vi "String - XML 2-Byte Decoding.vi"(0 "Number In (3-Bytes -24bits)":i32 format="%x", 3 "Error In":errorcluster) -> (7 "Output (\\ Format)":string, 8 "Output 16bits":i16=-30048 format="%04x", 10 "Error Out":errorcluster)   [LabVIEW 2013]
panel:
  out "YYYYYY  (6bits) 3":i32=2560 format="%024b"
  in  "Use Number In":bool=TRUE
  out "16bits":u32 format="%x"
  in  "String In (3-Byte Width)":string
  out "Swapped Bytes":i16=21152 format="%x"
  out "ZZZZZZ  (6bits) 3":i32=32 format="%024b"
  out "YYYYYY  (6bits) 2":i32=2560 format="%024b"
  out "XXXX  (4bits) 1":i32=327680 format="%024b"
  out "Output  (24bits)":i32=15043232 format="%024b"
  out "Input (21bits)":u32=21152 format="%021b"
  # "Otherwise, if the code point is less than 10000 (16) output the bitwise inclusive OR of bits 13 through 16 with EO16"
  # "E696 B0"
  # "B065"
  # "E58A A0"
  # "A052"
  # "E59DA1"
  # "6157"
  # "°e RaW"
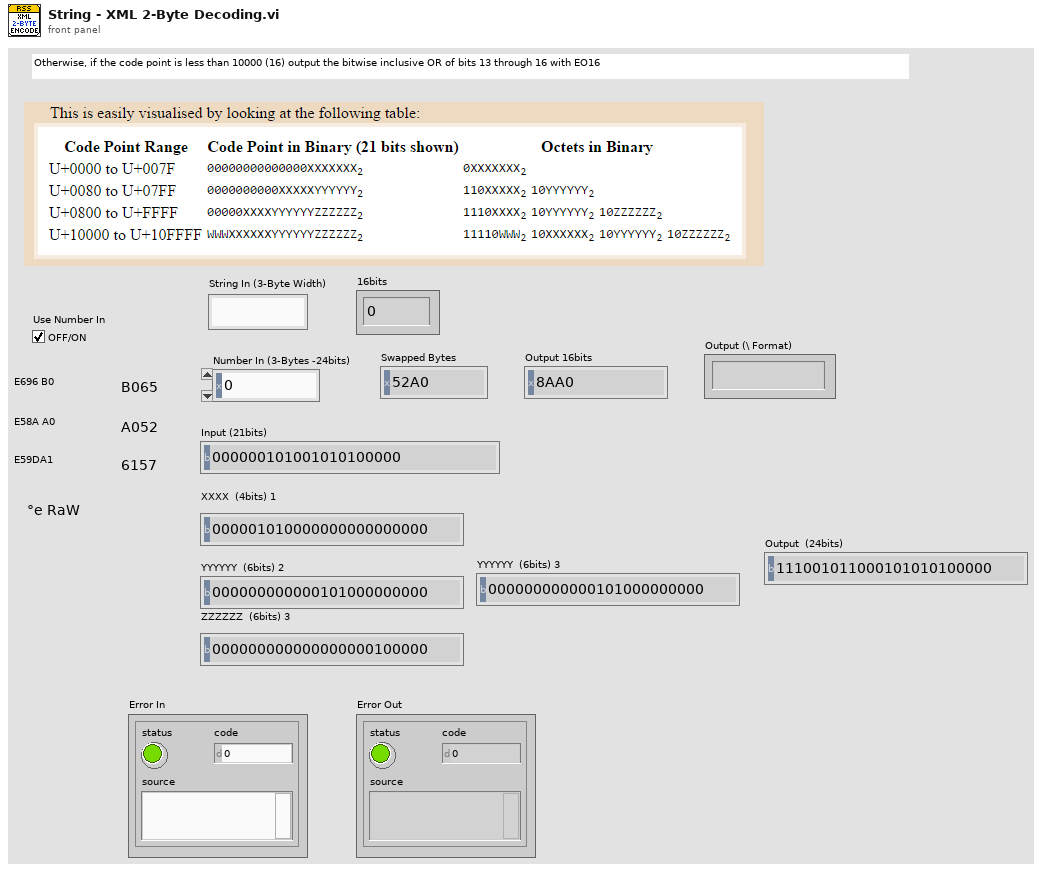
[diagram p1: front panel]
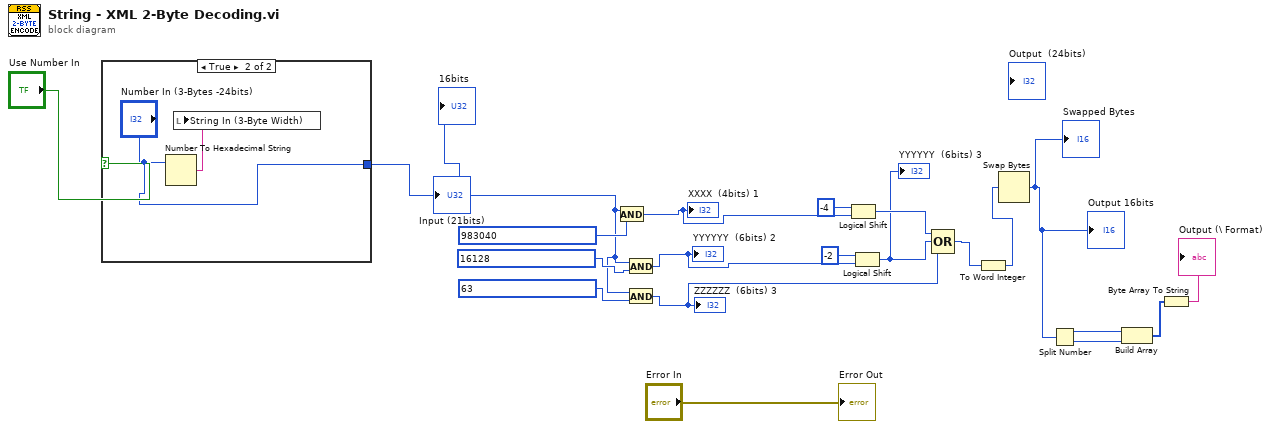
[diagram p0: block diagram]
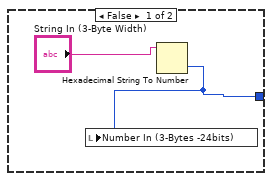
[diagram p2: hidden frame]
diagram:
  n1 = case shown="True" "Use Number In" {
    tunnel: [w21 "Number In (3-Bytes -24bits)"] -> w15
    frame False {
      n2 = Hexadecimal String To Number(string="String In (3-Byte Width)") -> (number=w21:u32)  [unwired: 2 in, 1 out]
      n3 = local write "Number In (3-Bytes -24bits)"(w21) -> ()
    }
    frame True {
      n4 = Number To Hexadecimal String(2:"Number In (3-Bytes -24bits)") -> (0:w24:string)  [unwired: 1 in]
      n5 = local write "String In (3-Byte Width)"(w24) -> ()
    }
  }
  "Input (21bits)" <- w15
  "16bits" <- w15
  n6 = And(x=w15, y=983040) -> (x .and. y?=w12:u32)
  "XXXX  (4bits) 1" <- w12
  n7 = And(x=w15, y=i16 16128) -> (x .and. y?=w14:u32)
  "YYYYYY  (6bits) 2" <- w14
  n8 = And(x=w15, y=i16 63) -> (x .and. y?=w9:u32)
  "ZZZZZZ  (6bits) 3" <- w9
  n9 = Logical Shift(y=i16 -4, x=w12) -> (x << y=w10:u32)
  n10 = Logical Shift(y=i16 -2, x=w14) -> (x << y=w6:u32)
  "YYYYYY  (6bits) 3" <- w6
  n11 = Compound Arithmetic op=OR(w10, w6, w9) -> (w8:u32)
  n12 = To Word Integer(number=w8) -> (16bit integer=w7:i16)
  n13 = Swap Bytes(anything=w7) -> (byte swapped=w4:i16)
  "Output 16bits" <- w4
  "Swapped Bytes" <- w4
  n14 = Split Number(x=w4) -> (hi(x)=w3:u8, lo(x)=w2:u8)
  n15 = Build Array(w3, w2) -> (w5:u8[])
  n16 = Byte Array To String(unsigned byte array=w5) -> (string=→"Output (\\ Format)":string)
  "Error Out" <- "Error In"
